vi "Add Part.vi"(7 "Sep (; )":string="; ", 10 "New Portion":string, 11 "String In":string) -> (3 "String":string)   [LabVIEW 2020, in "HTTP Utils.lvlib" / "Cookie.lvclass"]
uses:
  Cookie.lvclass
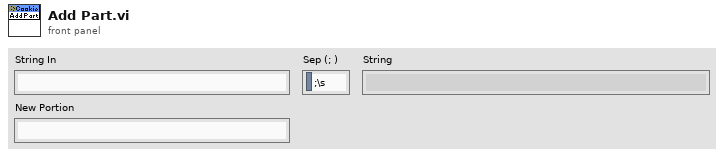
[diagram p1: front panel]
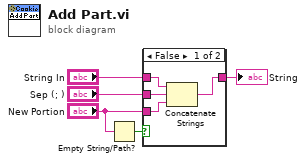
[diagram p0: block diagram]
diagram:
  n1 = Empty String/Path?(string/path="New Portion") -> (empty?=w5:bool)
  n2 = case shown="False" w5 {
    tunnel: "New Portion" -> [w7 _]
    tunnel: "String In" -> [w8 w10]
    tunnel: [w6 w10] -> w2
    tunnel: "Sep (; )" -> [w9 _]
    frame False {
      n3 = Concatenate Strings(w8, w9, w7) -> (w6:string)
    }
    frame True {
    }
  }
  "String" <- w2
